vi "UDP Dispatcher.vi"(0 "UDP port (0)":u16, 5 "use any port (F)":bool, 11 "error in":errorcluster) -> (15 "error out":errorcluster)   [LabVIEW 2014, in "AMC.lvlib"]
uses:
  AMC.lvlib
  Dispatcher State Variables.ctl
  FG Dispatcher Status Action.ctl
  <vilib>/NI/Tools/Keyed Array/Map String.vi
  <vilib>/NI/Tools/String/Get Case Matching.vi
  Globals.vi
  TCP handler.vi
  <vilib>/NI/Tools/Keyed Array/Tools_KeyedArray.lvlib
panel:
  in  "init complete":refnum<notifier>
  out "dispatcher error":errorcluster
  out "source process":string
  out "source host":string
  in  "stop":bool
  out "message string":string
  out "status":string
  # "Receive"
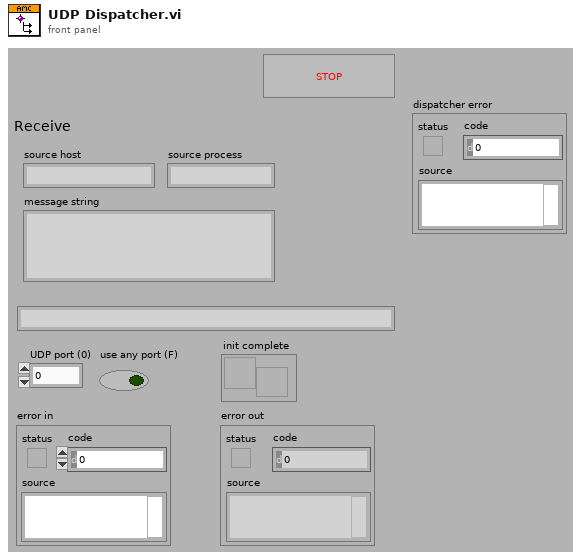
[diagram p1: front panel]
types:
  T1 = typedef "AMC.lvlib/FG Dispatcher Status Action.ctl" = enum16{"Get", "Force Init", "Close"}
  T2 = typedef "AMC.lvlib/Dispatcher State Variables.ctl" = cluster{"UDP port":u16}
  T3 = typedef "AMC.lvlib/Message Queue.ctl" = refnum<queue>
  T4 = typedef "AMC.lvlib/Message.ctl" = cluster{"name":string, "value":string, "attributes":T5, "receiver host":string, "receiver process":string, "source host":string, "source process":string, "priority message":bool, "acknowledge message":bool}
  T5 = typedef "Tools_KeyedArray.lvlib/KeyedArray.ctl" = cluster{"keys":string[], "values":string[]}
  T6 = typedef "AMC.lvlib/Queue Registry Properties.ctl" = cluster{"Name":string}
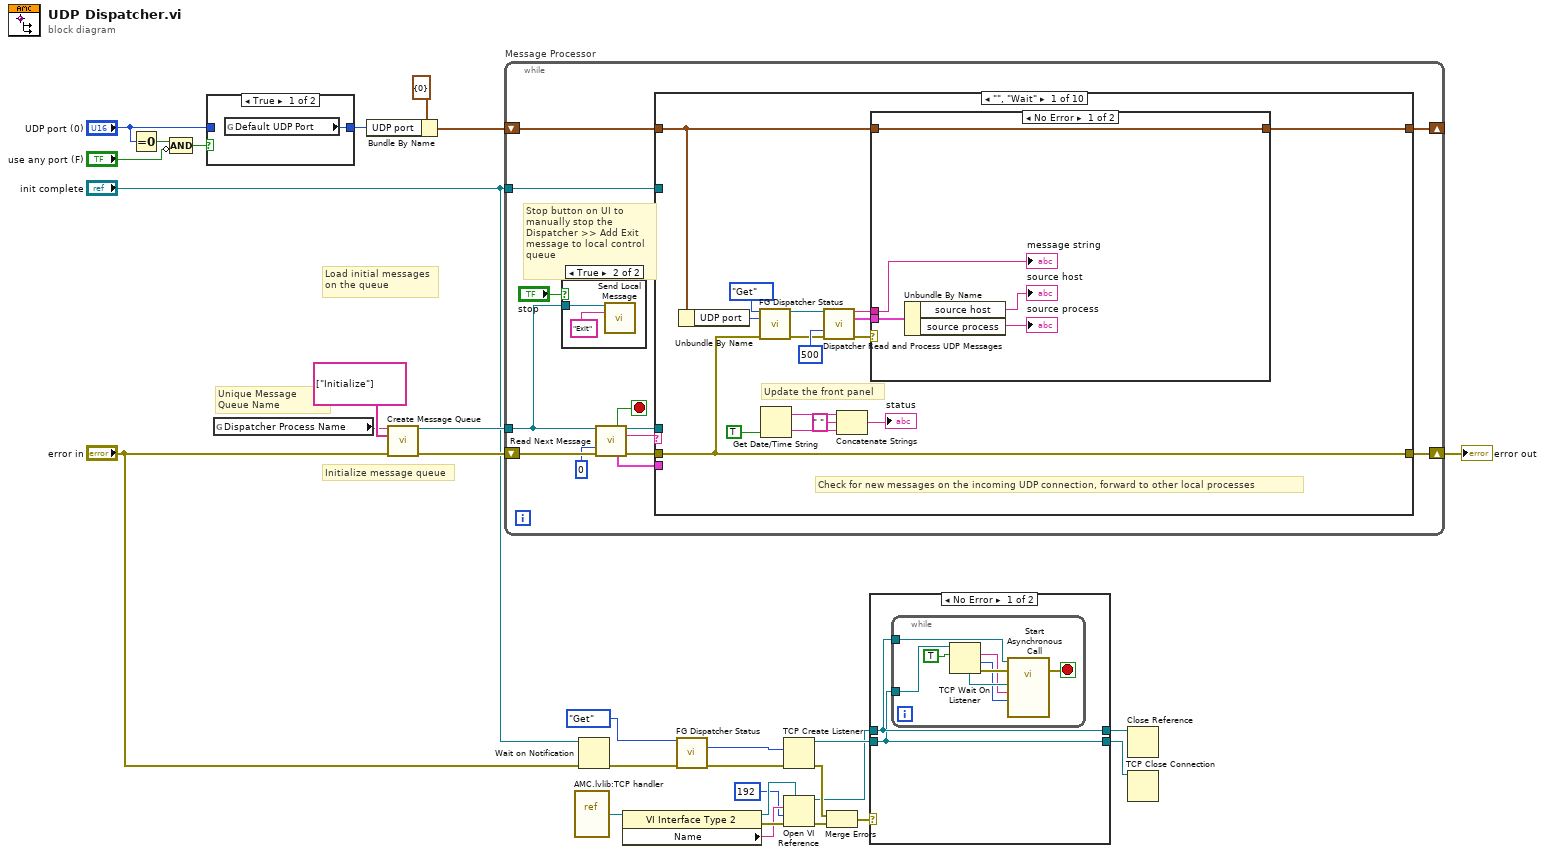
[diagram p0: block diagram]
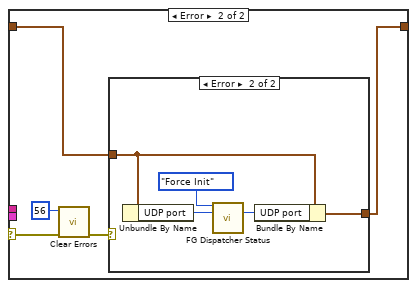
[diagram p5: hidden frame]
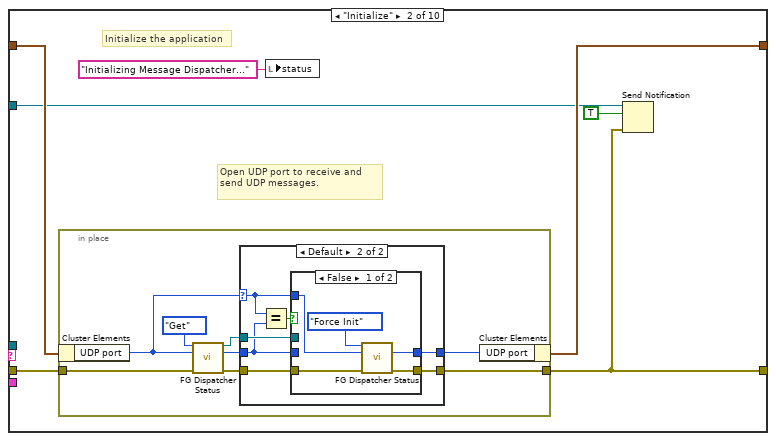
[diagram p7: hidden frame]
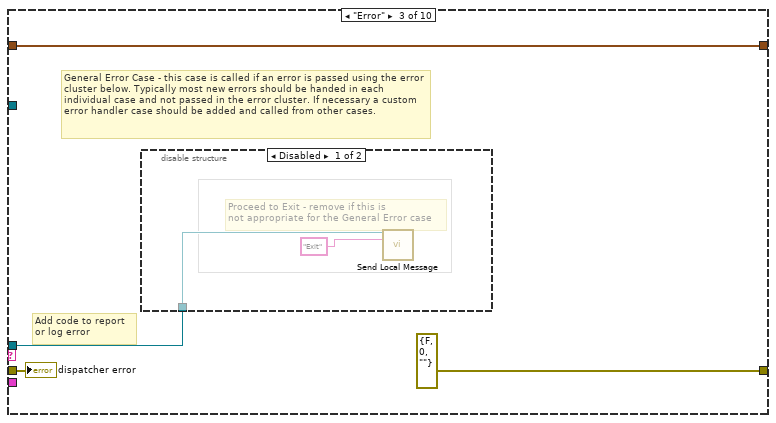
[diagram p10: hidden frame]
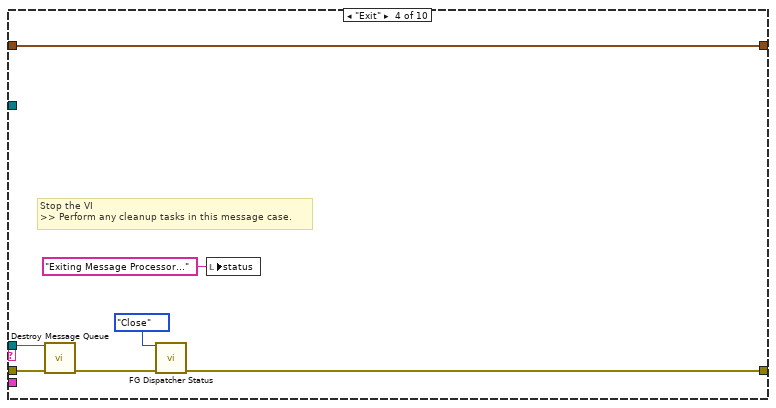
[diagram p12: hidden frame]
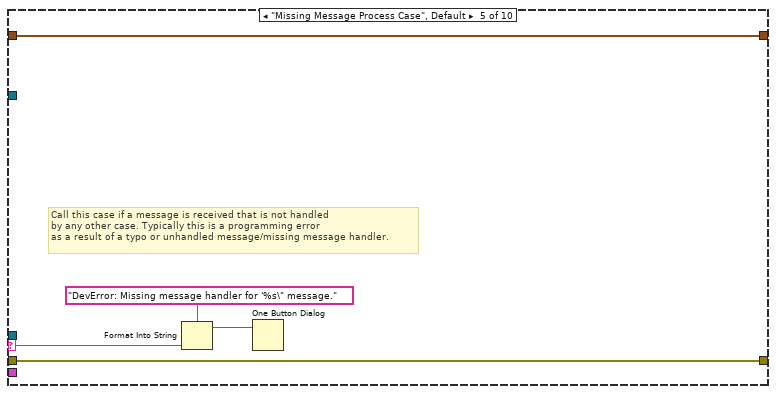
[diagram p13: hidden frame]
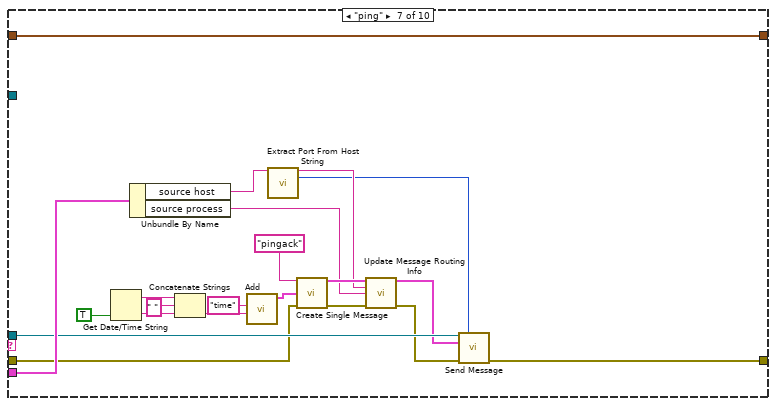
[diagram p15: hidden frame]
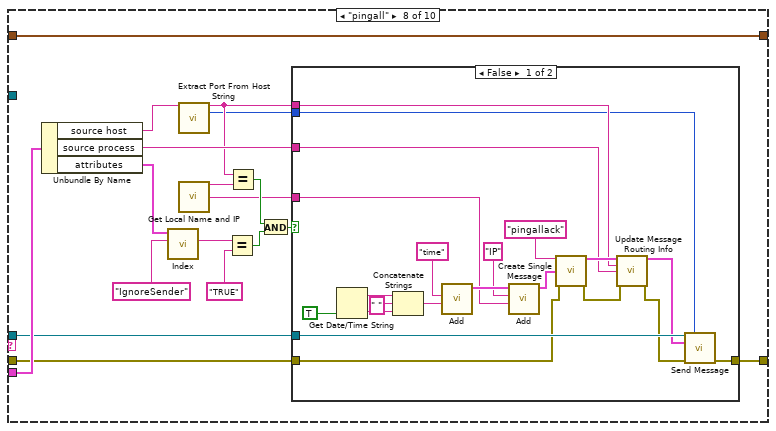
[diagram p16: hidden frame]
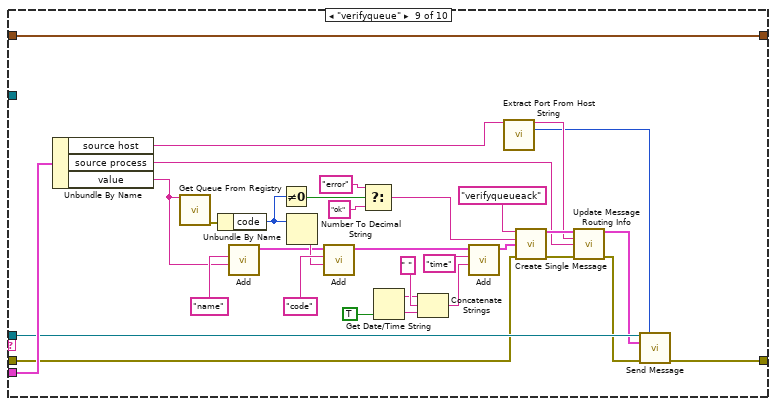
[diagram p18: hidden frame]
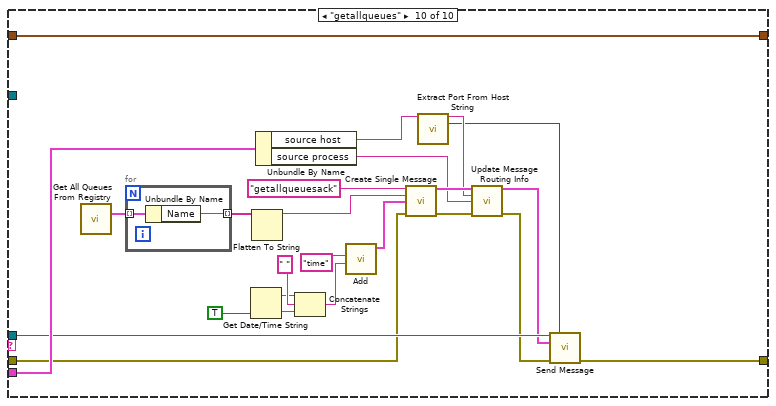
[diagram p19: hidden frame]
diagram:
  # "Initialize message queue"
  # "Unique Message Queue Name"
  # "Load initial messages\non the queue"
  n1 = Equal To 0?(x="UDP port (0)") -> (x = 0?=w22:bool)
  n2 = Compound Arithmetic op=AND(w22, invert "use any port (F)") -> (w20:bool)
  n3 = case shown="True" w20 {
    tunnel: [w31 w32] -> w23
    tunnel: "UDP port (0)" -> [_ w32]
    frame True {
      n4 = global read "Globals.vi" "Default UDP Port"() -> (w31:u16)
    }
    frame False {
    }
  }
  n5 = global read "Globals.vi" "Dispatcher Process Name"() -> (w27:string)
  n6 = Bundle By Name(cluster=T2 {"UDP port"=0} ("state variables"), "UDP port"=w23) -> (w25:T2)
  n7 = call "Create Message Queue.vi"("message queue name"=w27, "initial message names"=string[] ["Initialize"], "error in"="error in") -> ("message queue out"=w30:T3, "error out"=w29:errorcluster)  [unwired: 11 in]
  n8 = while "Message Processor" {
    shift-left: w29 -> [w41]
    shift-right: [w42] -> w24
    tunnel: w30 -> [w37]
    shift-left: w25 -> [w45]
    shift-right: [w36] -> _
    tunnel: "init complete" -> [w34]
    stop <- w39 stop-if-true
    # "Stop button on UI to\nmanually stop the\nDispatcher >> Add Exit\nmessage to local control\nqueue"
    n9 = case shown="True" "stop" {
      tunnel: w37 -> [_ w46]
      frame False {
      }
      frame True {
        n10 = call "Send Local Message.vi"("message queue in"=w46, "message name"="Exit") -> ()  [unwired: 11 in, 3 out]
      }
    }
    n11 = call "Read Next Message.vi"("message queue in"=w37, "timeout (1 ms)"=0 ("timeout (1ms)"), "error in"=w41) -> ("exit process?"=w39:bool, "message queue out"=w44:T3, "message name"=w40:string, "message"=w35:T4, "error out"=w43:errorcluster)  [unwired: 5 in, 3 out]
    n12 = case shown="\"\", \"Wait\"" w40 {
      selector: w40 -> [_ _ _ _ w126 _ _ _ _ _]
      tunnel: w45 -> [w48 w85 w114 w121 w128 w130 w151 w169 w224 w248]
      tunnel: w44 -> [_ _ w112 w122 _ _ w140 w156 w201 w236]
      tunnel: w43 -> [w53 w83 w111 w123 w127 w129 w136 w158 w197 w229]
      tunnel: [w53 w81 errorcluster {"status"=FALSE, "code"=0, "source"=""} ("error out") w117 w127 w129 w143 w157 w205 w239] -> w42
      tunnel: [w50 w84 w114 w121 w128 w130 w151 w169 w224 w248] -> w36
      tunnel: w35 -> [_ _ _ _ _ _ w150 w168 w223 w247]
      tunnel: w34 -> [_ w82 _ _ _ _ _ _ _ _]
      frame "", "Wait" {
        # "Check for new messages on the incoming UDP connection, forward to other local processes"
        # "Update the front panel"
        n13 = Unbundle By Name(w48) -> ("UDP port"=w49:u16)
        n14 = call "FG Dispatcher Status.vi"("action (Get)"=FG_Dispatcher_Status_Action."Get", "UDP port in (0)"=w49, "error in"=w53) -> ("UDP connection ID"=w51:refnum<k16>, "error out"=w52:errorcluster)  [unwired: 10 in, 1 out]
        n15 = Get Date/Time String(want seconds? (F)=TRUE) -> (date string=w63:string, time string=w62:string)  [unwired: 2 out]
        n16 = call "Dispatcher Read and Process UDP Messages.vi"("UDP conn ID"=w51, "timeout (10 ms)"=500, "error in"=w52) -> ("message string"=w58:string, "message"=w55:T4, "error out"=w57:errorcluster)  [unwired: 10 in]
        n17 = Concatenate Strings(w63, " " ("string"), w62) -> (→"status":string)
        n18 = case shown="No Error" w57 {
          selector: w57 -> [_ w73]
          tunnel: w58 -> [w68 _]
          tunnel: w55 -> [w67 _]
          tunnel: w48 -> [w64 w70]
          tunnel: [w64 w69] -> w50
          frame No Error {
            n19 = Unbundle By Name(w67) -> ("source host"=→"source host":string, "source process"=→"source process":string)
            "message string" <- w68
          }
          frame Error {
            n20 = call <vilib>:"Clear Errors.vi"("error in (no error)"=w73, "specific error code to clear (0: all)"=56) -> ("error out"=w71:errorcluster)  [unwired: 4 in, 1 out]
            n21 = case shown="Error" w71 {
              tunnel: w70 -> [w74 w78]
              tunnel: [w74 w75] -> w69
              frame No Error {
                # "just a timeout, no worries"
              }
              frame Error {
                n22 = Unbundle By Name(w78) -> ("UDP port"=w76:u16)
                n23 = call "FG Dispatcher Status.vi"("action (Get)"=FG_Dispatcher_Status_Action."Force Init", "UDP port in (0)"=w76) -> ("UDP port out"=w77:u16)  [unwired: 11 in, 2 out]
                n24 = Bundle By Name(cluster=w78, "UDP port"=w77) -> (w75:T2)
              }
            }
          }
        }
      }
      frame "Initialize" {
        # "Open UDP port to receive and send UDP messages."
        # "Initialize the application"
        n25 = in-place {
          in-place-border: w83 -> [w93]
          in-place-border: [w87] -> w81
          n26 = in-place-cluster #1(w85) -> ("UDP port"=w92:u16)
          n27 = call "FG Dispatcher Status.vi"("action (Get)"=FG_Dispatcher_Status_Action."Get", "UDP port in (0)"=w92, "error in"=w93) -> ("UDP connection ID"=w89:refnum<k16>, "UDP port out"=w91:u16, "error out"=w90:errorcluster)  [unwired: 10 in]
          n28 = case shown="Default" w92 {
            selector: w92 -> [_ w97]
            tunnel: w91 -> [w96 w99]
            tunnel: w90 -> [w95 w102]
            tunnel: w89 -> [_ w100]
            tunnel: [w96 w98] -> w88
            tunnel: [w95 w101] -> w87
            frame 0 {
            }
            frame Default {
              n29 = Equal?(x=w97, y=w99) -> (x = y?=w103:bool)
              n30 = case shown="False" w103 {
                tunnel: w102 -> [w107 w110]
                tunnel: [w106 w110] -> w101
                tunnel: w100 -> [_ _]
                tunnel: w99 -> [_ w109]
                tunnel: [w104 w109] -> w98
                tunnel: w97 -> [w105 _]
                frame False {
                  n31 = call "FG Dispatcher Status.vi"("action (Get)"=FG_Dispatcher_Status_Action."Force Init", "UDP port in (0)"=w105, "error in"=w107) -> ("UDP port out"=w104:u16, "error out"=w106:errorcluster)  [unwired: 10 in, 1 out]
                }
                frame True {
                }
              }
            }
          }
          n32 = in-place-cluster #1("UDP port"=w88) -> (w84:T2)
        }
        n33 = local write "status"("Initializing Message Dispatcher..." ("message")) -> ()
        n34 = Send Notification(notification=TRUE, notifier=w82, error in (no error)=w81) -> ()  [unwired: 2 out]
      }
      frame "Error" {
        # "Add code to report\nor log error"
        # "General Error Case - this case is called if an error is passed using the error cluster below. Typically most new errors should be handed in each individual case and not passed in the error cluster. If necessary a custom error handler case should be added and called from other cases."
        n35 = disable-structure shown="Disabled" {
          disable-tunnel: w112 -> [w116 _]
          frame Disabled {
            # "Proceed to Exit - remove if this is\nnot appropriate for the General Error case"
            n36 = call "Send Local Message.vi"("message queue in"=w116, "message name"="Exit") -> ()  [unwired: 11 in, 3 out]
          }
          frame Enabled {
          }
        }
        "dispatcher error" <- w111
      }
      frame "Exit" {
        # "Stop the VI\n>> Perform any cleanup tasks in this message case."
        n37 = call "Destroy Message Queue.vi"("message queue in"=w122, "error in"=w123) -> ("error out"=w118:errorcluster)  [unwired: 11 in, 2 out]
        n38 = call "FG Dispatcher Status.vi"("action (Get)"=FG_Dispatcher_Status_Action."Close", "error in"=w118) -> ("error out"=w117:errorcluster)  [unwired: 11 in, 2 out]
        n39 = local write "status"("Exiting Message Processor..." ("button name (\"OK\")")) -> ()
      }
      frame "Missing Message Process Case", Default {
        # "Call this case if a message is received that is not handled \nby any other case. Typically this is a programming error\nas a result of a typo or unhandled message/missing message handler."
        n40 = Format Into String(format string="DevError: Missing message handler for '%s\" message." ("message"), w126) -> (resulting string=w124:string)  [unwired: 2 in, 1 out]
        n41 = One Button Dialog(message=w124) -> ()  [unwired: 2 out]
      }
      frame "**** Message Dispatcher Service Functions ****" {
      }
      frame "ping" {
        n42 = Get Date/Time String(want seconds? (F)=TRUE) -> (date string=w149:string, time string=w148:string)  [unwired: 2 out]
        n43 = Unbundle By Name(w150) -> ("source host"=w133:string, "source process"=w138:string)
        n44 = Concatenate Strings(w149, " ", w148) -> (w146:string)
        n45 = call <vilib>:"Add.vi"("value"=w146, "key"="time") -> ("array out"=w141:T5)  [unwired: 2 in, 3 out]
        n46 = call "Extract Port From Host String.vi"("host in"=w133) -> ("host out"=w132:string, "port"=w131:u16)  [unwired: 12 in, 1 out]
        n47 = call "Create Single Message.vi"("name"="pingack" ("Name"), "attributes"=w141, "error in"=w136) -> ("message"=w139:T4, "error out"=w137:errorcluster)  [unwired: 11 in]
        n48 = call "Update Message Routing Info.vi"("message"=w139, "receiver host (\"\")"=w132, "receiver process (\"\")"=w138, "error in"=w137) -> ("message"=w135:T4, "error out"=w134:errorcluster)  [unwired: 10 in]
        n49 = call "Send Message.vi"("message queue in"=w140, "receiver port"=w131, "message"=w135, "error in"=w134) -> ("error out"=w143:errorcluster)  [unwired: 9 in, 2 out]
      }
      frame "pingall" {
        n50 = Unbundle By Name(w168) -> ("source host"=w154:string, "source process"=w163:string, "attributes"=w167:T5)
        n51 = call <vilib>:"Index.vi"("key"="IgnoreSender", "array in"=w167) -> ("value"=w165:string)  [unwired: 2 in, 3 out]
        n52 = call "Extract Port From Host String.vi"("host in"=w154) -> ("host out"=w153:string, "port"=w152:u16)  [unwired: 12 in, 1 out]
        n53 = call "Get Local Name and IP.vi"() -> ("name"=w159:string, "IP address"=w155:string)  [unwired: 12 in, 2 out]
        n54 = Equal?(x=w165, y="TRUE" ("x")) -> (x = y?=w162:bool)
        n55 = Equal?(x=w153, y=w159) -> (x = y?=w161:bool)
        n56 = And(x=w161, y=w162) -> (x .and. y?=w160:bool)
        n57 = case shown="False" w160 {
          tunnel: w153 -> [w176 _]
          tunnel: w163 -> [w175 _]
          tunnel: w155 -> [w182 _]
          tunnel: w158 -> [w173 w191]
          tunnel: [w181 w191] -> w157
          tunnel: w156 -> [w178 _]
          tunnel: w152 -> [w170 _]
          frame False {
            n58 = Get Date/Time String(want seconds? (F)=TRUE) -> (date string=w190:string, time string=w189:string)  [unwired: 2 out]
            n59 = Concatenate Strings(w190, " ", w189) -> (w187:string)
            n60 = call <vilib>:"Add.vi"("value"=w187, "key"="time") -> ("array out"=w184:T5)  [unwired: 2 in, 3 out]
            n61 = call <vilib>:"Add.vi"("value"=w182, "key"="IP", "array in"=w184) -> ("array out"=w179:T5)  [unwired: 1 in, 3 out]
            n62 = call "Create Single Message.vi"("name"="pingallack" ("Name"), "attributes"=w179, "error in"=w173) -> ("message"=w177:T4, "error out"=w174:errorcluster)  [unwired: 11 in]
            n63 = call "Update Message Routing Info.vi"("message"=w177, "receiver host (\"\")"=w176, "receiver process (\"\")"=w175, "error in"=w174) -> ("message"=w172:T4, "error out"=w171:errorcluster)  [unwired: 10 in]
            n64 = call "Send Message.vi"("message queue in"=w178, "receiver port"=w170, "message"=w172, "error in"=w171) -> ("error out"=w181:errorcluster)  [unwired: 9 in, 2 out]
          }
          frame True {
            # "Do not respond if the PingAll request was sent by this system."
          }
        }
      }
      frame "verifyqueue" {
        n65 = Unbundle By Name(w223) -> ("source host"=w194:string, "source process"=w198:string, "value"=w207:string)
        n66 = call "Get Queue From Registry.vi"("name"=w207) -> ("error out"=w206:errorcluster)  [unwired: 13 in, 1 out]
        n67 = Unbundle By Name(w206) -> ("code"=w218:i32)
        n68 = call <vilib>:"Add.vi"("value"=w207, "key"="name") -> ("array out"=w220:T5)  [unwired: 2 in, 3 out]
        n69 = Not Equal To 0?(x=w218) -> (x != 0?=w217:bool)
        n70 = Number To Decimal String(number=w218) -> (decimal integer string=w221:string)  [unwired: 1 out]
        n71 = call <vilib>:"Add.vi"("value"=w221, "key"="code", "array in"=w220) -> ("array out"=w208:T5)  [unwired: 1 in, 3 out]
        n72 = Select(t="error", s=w217, f="ok") -> (s? t:f=w203:string)
        n73 = Get Date/Time String(want seconds? (F)=TRUE) -> (date string=w212:string, time string=w211:string)  [unwired: 2 out]
        n74 = Concatenate Strings(w212, " ", w211) -> (w210:string)
        n75 = call <vilib>:"Add.vi"("value"=w210, "key"="time", "array in"=w208) -> ("array out"=w202:T5)  [unwired: 1 in, 3 out]
        n76 = call "Extract Port From Host String.vi"("host in"=w194) -> ("host out"=w193:string, "port"=w192:u16)  [unwired: 12 in, 1 out]
        n77 = call "Create Single Message.vi"("name"="verifyqueueack" ("Name"), "value"=w203, "attributes"=w202, "error in"=w197) -> ("message"=w200:T4, "error out"=w195:errorcluster)  [unwired: 10 in]
        n78 = call "Update Message Routing Info.vi"("message"=w200, "receiver host (\"\")"=w193, "receiver process (\"\")"=w198, "error in"=w195) -> ("message"=w199:T4, "error out"=w196:errorcluster)  [unwired: 10 in]
        n79 = call "Send Message.vi"("message queue in"=w201, "receiver port"=w192, "message"=w199, "error in"=w196) -> ("error out"=w205:errorcluster)  [unwired: 9 in, 2 out]
      }
      frame "getallqueues" {
        n80 = call "Get All Queues From Registry.vi"() -> ("all properties"=w240:T6[])  [unwired: 12 in, 3 out]
        n81 = for {
          tunnel: w240 -> [w250] mode=indexing
          tunnel: [w249] -> w235 mode=indexing
          n82 = Unbundle By Name(w250) -> ("Name"=w249:string)
        }
        n83 = Get Date/Time String(want seconds? (F)=TRUE) -> (date string=w244:string, time string=w243:string)  [unwired: 2 out]
        n84 = Flatten To String(anything=w235) -> (data string=w234:string)  [unwired: 3 in, 2 out]
        n85 = Unbundle By Name(w247) -> ("source host"=w227:string, "source process"=w231:string)
        n86 = Concatenate Strings(w244, " ", w243) -> (w242:string)
        n87 = call <vilib>:"Add.vi"("value"=w242, "key"="time") -> ("array out"=w237:T5)  [unwired: 2 in, 3 out]
        n88 = call "Create Single Message.vi"("name"="getallqueuesack" ("Name"), "value"=w234, "attributes"=w237, "error in"=w229) -> ("message"=w233:T4, "error out"=w230:errorcluster)  [unwired: 10 in]
        n89 = call "Extract Port From Host String.vi"("host in"=w227) -> ("host out"=w226:string, "port"=w225:u16)  [unwired: 12 in, 1 out]
        n90 = call "Update Message Routing Info.vi"("message"=w233, "receiver host (\"\")"=w226, "receiver process (\"\")"=w231, "error in"=w230) -> ("message"=w232:T4, "error out"=w228:errorcluster)  [unwired: 10 in]
        n91 = call "Send Message.vi"("message queue in"=w236, "receiver port"=w225, "message"=w232, "error in"=w228) -> ("error out"=w239:errorcluster)  [unwired: 9 in, 2 out]
      }
    }
  }
  "error out" <- w24
  n92 = vi-ref "AMC.lvlib:TCP handler.vi"() -> (w8:refnum<vi>)
  n93 = Wait on Notification(notifier="init complete", error in (no error)="error in") -> (error out=w15:errorcluster)  [unwired: 2 in, 3 out]
  n94 = property class="VI Interface Type 2"(reference=w8) -> (reference out=w6:refnum<vi>, error out=w9:errorcluster, "Name"=w7:string)  [unwired: 1 in]
  n95 = call "FG Dispatcher Status.vi"("action (Get)"=FG_Dispatcher_Status_Action."Get", "error in"=w15) -> ("UDP port out"=w13:u16, "error out"=w14:errorcluster)  [unwired: 11 in, 1 out]
  n96 = TCP Create Listener(8:w14, 10:w13) -> (0:w11:errorcluster, 3:w12:refnum<k5>)  [unwired: 3 in, 1 out]
  n97 = Open VI Reference(type specifier VI Refnum (for type only)=w6, vi path=w7, options=192, error in (no error)=w9) -> (vi reference=w3:refnum<vi>, error out=w4:errorcluster)  [unwired: 2 in]
  n98 = Merge Errors(w11, w4) -> (w10:errorcluster)
  n99 = case shown="No Error" w10 {
    tunnel: w12 -> [w251 w261]
    tunnel: w3 -> [w252 w262]
    tunnel: [w252 w262] -> w2
    tunnel: [w251 w261] -> w1
    frame No Error {
      n100 = while {
        tunnel: w251 -> [w260]
        tunnel: w252 -> [w256]
        stop <- w257 stop-if-true
        n101 = TCP Wait On Listener(10:TRUE ("resolve remote address (T)"), 11:w260) -> (0:w258:errorcluster, 1:w253:u16, 2:w254:string, 4:w255:refnum<k5>)  [unwired: 2 in, 1 out]
        n102 = call-by-ref "Start Asynchronous Call"(reference=w256, error in=w258, "remote port"=w253, "remote address"=w254, "connection ID"=w255) -> (error out=w257:errorcluster)  [unwired: 9 in, 1 out]
      }
    }
    frame Error {
    }
  }
  n103 = Close Reference(reference=w2) -> ()  [unwired: 1 in, 1 out]
  n104 = TCP Close Connection(connection ID=w1) -> ()  [unwired: 2 in, 2 out]
